vi "Laufschrift.vi"() -> ()   [LabVIEW 2010]
panel:
  in  "laufschrift":bool
  in  "BG color(transparent)":u32(colorbox)=16777216 caption="Hintergrundfarbe(Transparent)"
  in  "text color(black)":u32(colorbox) caption="Textfarbe(Schwarz)"
  in  "origin":cluster{"x":i16, "y":i16}={"x"=0, "y"=1} caption="Ursprung"
  in  "filename without extension":string caption="Text"
  out "bild-nahme":picture
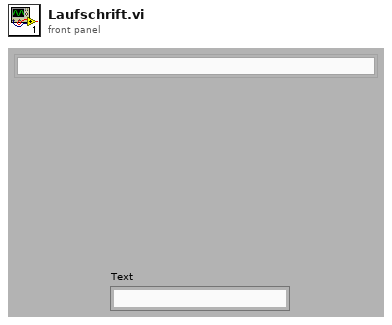
[diagram p1: front panel]
types:
  T1 = cluster{"horizontal":enum16{"left", "center", "right"}, "vertical":enum16{"top", "center", "bottom"}}
  T2 = enum16{"None", "Stacked", "Clockwise", "Counterclockwise"}
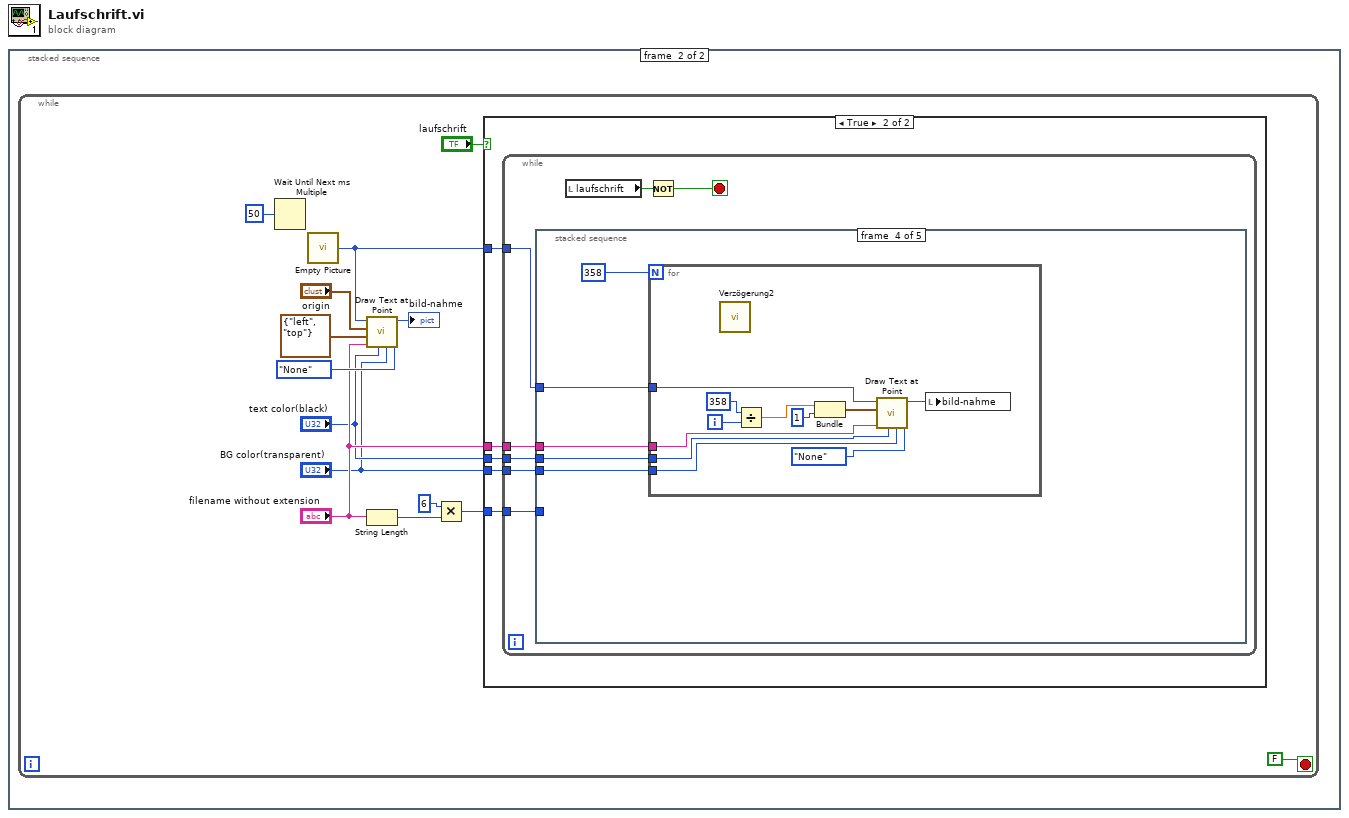
[diagram p0: block diagram]
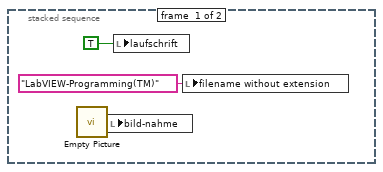
[diagram p2: hidden frame]
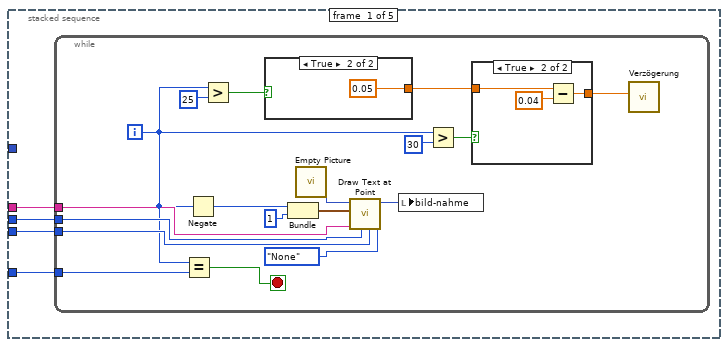
[diagram p4: hidden frame]
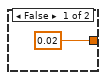
[diagram p6: hidden frame]
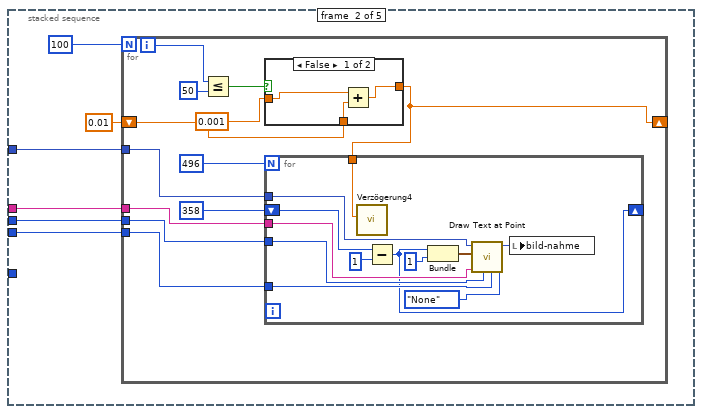
[diagram p7: hidden frame]
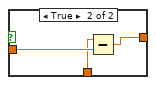
[diagram p8: hidden frame]
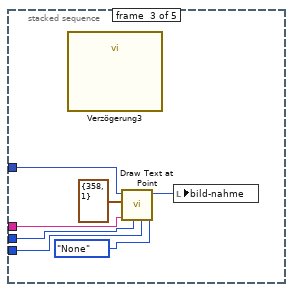
[diagram p9: hidden frame]
diagram:
  n1 = stacked-sequence {
    frame #0 {
      n2 = call "Empty Picture"() -> ("empty picture"=w3:picture)
      n3 = local write "bild-nahme"(w3) -> ()
      n4 = local write "laufschrift"(TRUE ("laufschrift")) -> ()
      n5 = local write "filename without extension"("LabVIEW-Programming(TM)" ("filename without extension")) -> ()
    }
    frame #1 {
      n6 = while {
        stop <- FALSE stop-if-true
        n7 = Wait Until Next ms Multiple(millisecond multiple=50) -> ()  [unwired: 1 out]
        n8 = call "Empty Picture"() -> ("empty picture"=w8:picture)
        n9 = call <vilib>:"Draw Text at Point.vi"("text orientation"=T2."None", "BG color(transparent)"="BG color(transparent)", "text color(black)"="text color(black)", "text"="filename without extension", "alignment(left, top)"=T1 {"horizontal"=enum."left", "vertical"=enum."top"}, "origin"="origin", "picture"=w8) -> ("new picture"=→"bild-nahme":picture)  [unwired: 2 in, 2 out]
        n10 = String Length(string="filename without extension") -> (length=w4:i32)
        n11 = Multiply(x=6, y=w4) -> (x*y=w11:i32)
        n12 = case shown="TRUE" "laufschrift" {
          tunnel: w11 -> [_ w22]
          tunnel: "filename without extension" -> [_ w21]
          tunnel: w8 -> [_ w20]
          tunnel: "text color(black)" -> [_ w19]
          tunnel: "BG color(transparent)" -> [_ w18]
          frame False {
          }
          frame True {
            n13 = while {
              tunnel: w22 -> [w29]
              tunnel: w21 -> [w26]
              tunnel: w20 -> [w28]
              tunnel: w19 -> [w24]
              tunnel: w18 -> [w23]
              stop <- w25 stop-if-true
              n14 = stacked-sequence {
                tunnel: w29 -> [w33 _ _ _ _]
                tunnel: w26 -> [w32 w61 w97 w103 _]
                tunnel: w28 -> [_ w60 w99 w105 _]
                tunnel: w24 -> [w31 w62 w94 w101 _]
                tunnel: w23 -> [w30 w63 w95 w102 _]
                frame #0 {
                  n15 = while {
                    tunnel: w33 -> [w49]
                    tunnel: w32 -> [w43]
                    tunnel: w31 -> [w42]
                    tunnel: w30 -> [w41]
                    i -> [w37]
                    stop <- w48 stop-if-true
                    n16 = Equal?(x=w37, y=w49) -> (x = y?=w48:bool)
                    n17 = Negate(x=w37) -> (-x=w50:i32)
                    n18 = Greater?(x=w37, y=25) -> (0:w39:bool)
                    n19 = case shown="TRUE" w39 {
                      tunnel: [0.02 ("Delay Time (s)") 0.05 ("Delay Time (s)")] -> w35
                      frame False {
                      }
                      frame True {
                      }
                    }
                    n20 = Bundle(w50, 1) -> (w47:cluster{i32, i32})  [unwired: 1 out]
                    n21 = call "Empty Picture"() -> ("empty picture"=w46:picture)
                    n22 = call <vilib>:"Draw Text at Point.vi"("text orientation"=T2."None", "BG color(transparent)"=w41, "text color(black)"=w42, "text"=w43, "origin"=w47, "picture"=w46) -> ("new picture"=w45:picture)  [unwired: 3 in, 2 out]
                    n23 = local write "bild-nahme"(w45) -> ()
                    n24 = Greater?(x=w37, y=30) -> (0:w36:bool)
                    n25 = case shown="TRUE" w36 {
                      tunnel: w35 -> [w52 w55]
                      tunnel: [w52 w53] -> w34
                      frame False {
                      }
                      frame True {
                        n26 = Subtract(x=w55, y=0.04) -> (x-y=w53:dbl)
                      }
                    }
                    n27 = call "Verzögerung"("Delay Time (s)"=w34) -> ()  [unwired: 1 in, 10 out]
                  }
                }
                frame #1 {
                  n28 = for {
                    N: 100 -> [_]
                    tunnel: w63 -> [w74]
                    tunnel: w62 -> [w73]
                    tunnel: w61 -> [w72]
                    tunnel: w60 -> [w71]
                    shift-right: [w64] -> _
                    shift-left: 0.01 -> [w65]
                    i -> [w69]
                    n29 = Less Or Equal?(x=w69, y=50) -> (x <= y?=w67:bool)
                    n30 = case shown="FALSE" w67 {
                      tunnel: 0.001 -> [w78 w81]
                      tunnel: [w76 w80] -> w64
                      tunnel: w65 -> [w77 w79]
                      frame False {
                        n31 = Add(x=w78, y=w77) -> (x+y=w76:dbl)
                      }
                      frame True {
                        n32 = Subtract(x=w79, y=w81) -> (x-y=w80:dbl)
                      }
                    }
                    n33 = for {
                      N: 496 -> [_]
                      tunnel: w72 -> [w86]
                      tunnel: w74 -> [w89]
                      tunnel: w73 -> [w88]
                      tunnel: w71 -> [w87]
                      shift-right: [w83] -> _
                      shift-left: 358 -> [w85]
                      tunnel: w64 -> [w82]
                      n34 = call "Verzögerung4"("Delay Time (s)"=w82) -> ()  [unwired: 1 in, 10 out]
                      n35 = Subtract(x=w85, y=1) -> (x-y=w83:i32)
                      n36 = Bundle(w83, 1) -> (w90:cluster{i32, i32})  [unwired: 1 out]
                      n37 = call <vilib>:"Draw Text at Point.vi"("text orientation"=T2."None", "BG color(transparent)"=w89, "text color(black)"=w88, "text"=w86, "origin"=w90, "picture"=w87) -> ("new picture"=w93:picture)  [unwired: 3 in, 2 out]
                      n38 = local write "bild-nahme"(w93) -> ()
                    }
                  }
                }
                frame #2 {
                  n39 = call "Verzögerung3"() -> ()  [unwired: 2 in, 10 out]
                  n40 = call <vilib>:"Draw Text at Point.vi"("text orientation"=T2."None", "BG color(transparent)"=w95, "text color(black)"=w94, "text"=w97, "origin"=cluster{"x":i16, "y":i16} {"x"=358, "y"=1}, "picture"=w99) -> ("new picture"=w100:picture)  [unwired: 3 in, 2 out]
                  n41 = local write "bild-nahme"(w100) -> ()
                }
                frame #3 {
                  n42 = for {
                    N: 358 -> [_]
                    tunnel: w105 -> [w114]
                    tunnel: w103 -> [w108]
                    tunnel: w102 -> [w107]
                    tunnel: w101 -> [w106]
                    i -> [w113]
                    n43 = call "Verzögerung2"() -> ()  [unwired: 2 in, 10 out]
                    n44 = Divide(x=358, y=w113) -> (x/y=w109:dbl)
                    n45 = Bundle(w109, 1) -> (w111:cluster{dbl, i32})  [unwired: 1 out]
                    n46 = call <vilib>:"Draw Text at Point.vi"("text orientation"=T2."None", "BG color(transparent)"=w107, "text color(black)"=w106, "text"=w108, "origin"=w111, "picture"=w114) -> ("new picture"=w116:picture)  [unwired: 3 in, 2 out]
                    n47 = local write "bild-nahme"(w116) -> ()
                  }
                }
                frame #4 {
                }
              }
              n48 = local read "laufschrift"() -> (w27:bool)
              n49 = Not(x=w27) -> (.not. x?=w25:bool)
            }
          }
        }
      }
    }
  }
